vi "StandardEngineUI.vi"() -> ()   [LabVIEW 2013, in "Standard Engine Editor Node.lvclass"]
doc: "This VI creates a view for the Standard Engine Configuration class using the CEF."
uses:
  Standard Engine Editor Node.lvclass
  <vilib>/NI/Configuration Framework/Node/NodeRef.ctl
  <vilib>/NI/Configuration Framework/Node/NISE_CEF_Node.lvclass
  <vilib>/NI/AMC/Message Queue.ctl
  <vilib>/NI/AMC/Message.ctl
  <vilib>/NI/Tools/Keyed Array/KeyedArray.ctl
  <vilib>/NI/Configuration Framework/Node/UserEventRef.ctl
  <vilib>/NI/Configuration Framework/Controls/EventCluster.ctl
  Execution Engine/Configuration/Supported Timing Sources.ctl
  Processor Assignment Mode.ctl
  <vilib>/NI/Configuration Framework/Node/RefreshUIEvent.ctl
  <vilib>/NI/Configuration Framework/Node/CacheState.ctl
  <vilib>/NI/Configuration Framework/Node/StopEvent.ctl
  <vilib>/NI/Configuration Framework/Node/NodeChangeEvent.ctl
  Execution Engine/Configuration/timing reporting tags.ctl
  Execution Engine/Configuration/error options.ctl
  Execution Engine/Configuration/pre-execution timing tags.ctl
  <vilib>/Utility/miscctls.llb/LVPositionTypeDef.ctl
  <vilib>/NI/DCAF/Tag Editor Core/Configuration Editor/Classes/Engine Parent/Engine Parent Editor Node.lvclass
  Standard Engine Editor Node.lvclass/Standard Engine Editor Node.ctl
  Execution Engine/Configuration/Standard Engine Configuration.lvclass/Standard Engine Configuration.ctl
  Execution Engine/Configuration/Module Decimation.ctl
  Execution Engine/Runtime/error responses.ctl
  Execution Engine/Configuration/Write Timing Source Type.vi
  Execution Engine/Configuration/Write Master Timing Module.vi
  Execution Engine/Configuration/Write Processor.vi
  Execution Engine/Configuration/Read Processor.vi
  Execution Engine/Configuration/Read Timing Source Type.vi
  <vilib>/NI/DCAF/Tag Editor Core/Configuration Editor/Classes/Engine Parent/Read Name.vi
  <vilib>/NI/Configuration Framework/serializable configuration/get alias.vi
  Execution Engine/Configuration/Write Timing Source dt.vi
  Execution Engine/Configuration/Find Module Specific Config.vi
  <vilib>/NI/Configuration Framework/error generator/NISE_error generator.vi
  Execution Engine/Configuration/Read Timing Source dt.vi
  <vilib>/NI/DCAF UI Toolkit/Controls/DCAF UI Elements.lvlib
  Execution Engine/Configuration/Standard Engine Configuration.lvclass
  <vilib>/NI/Configuration Framework/serializable configuration/NISE_CEF_serializable configuration.lvclass
  <vilib>/NI/Tools/Keyed Array/Tools_KeyedArray.lvlib
  <vilib>/NI/AMC/AMC.lvlib
  <vilib>/NI/Configuration Framework/NISE_CEF_TreeControl.lvlib
panel:
  in  "node change":T1
  in  "stop event":T2
  in  "cache state":T3
  in  "refresh UI":T4
  in  "Tab Control":enum32{"Engine Settings", "Module Settings"}(tab)
  out "Pre-Execution Timing Tags":T5
  in  "Create Pre-Execution Timing Tags?":bool=TRUE
  in  "Create Timing Report Tags?":bool
  in  "Module Timing Source":i32(listbox)
  in  "Engine Name":string
  in  "Timing Source dt":u32=5000
  in  "Timing Source Type":T6=enum."1 kHz Clock"
  in  "Procesor Assignment":i32 min=0
  in  "Mode":T7
  in  "Warning Message":string="This timing source is not deterministic."
  out "Timing Reporting":T8={"late index (bool)"="_stdeng_late", "late count index (U32)"="_stdeng_latecount", "current dt ns(U64)"="_stdeng_iteratedt", "last exec time ns(U64)"="_stdeng_exectime"}
  in  "Offset":u16
  in  "Decimation":u16=1 min=1
  in  "Create Error Tag?":bool
  out "error tag":string
  in  "Module to Configure":i32(listbox)
  in  "Execution Order (low to high)":i32
  in  "Execute Asynchronously?":bool
  in  "Recoverable":T9
  in  "Critical":T9
  in  "Trivial":T9
  in  "Unknown":T9
  in  "user event":T10
  in  "main queue":T11
  in  "node ref":T12
  # "Processor Assignment"
  # "Timing Information"
  # "Error Actions"
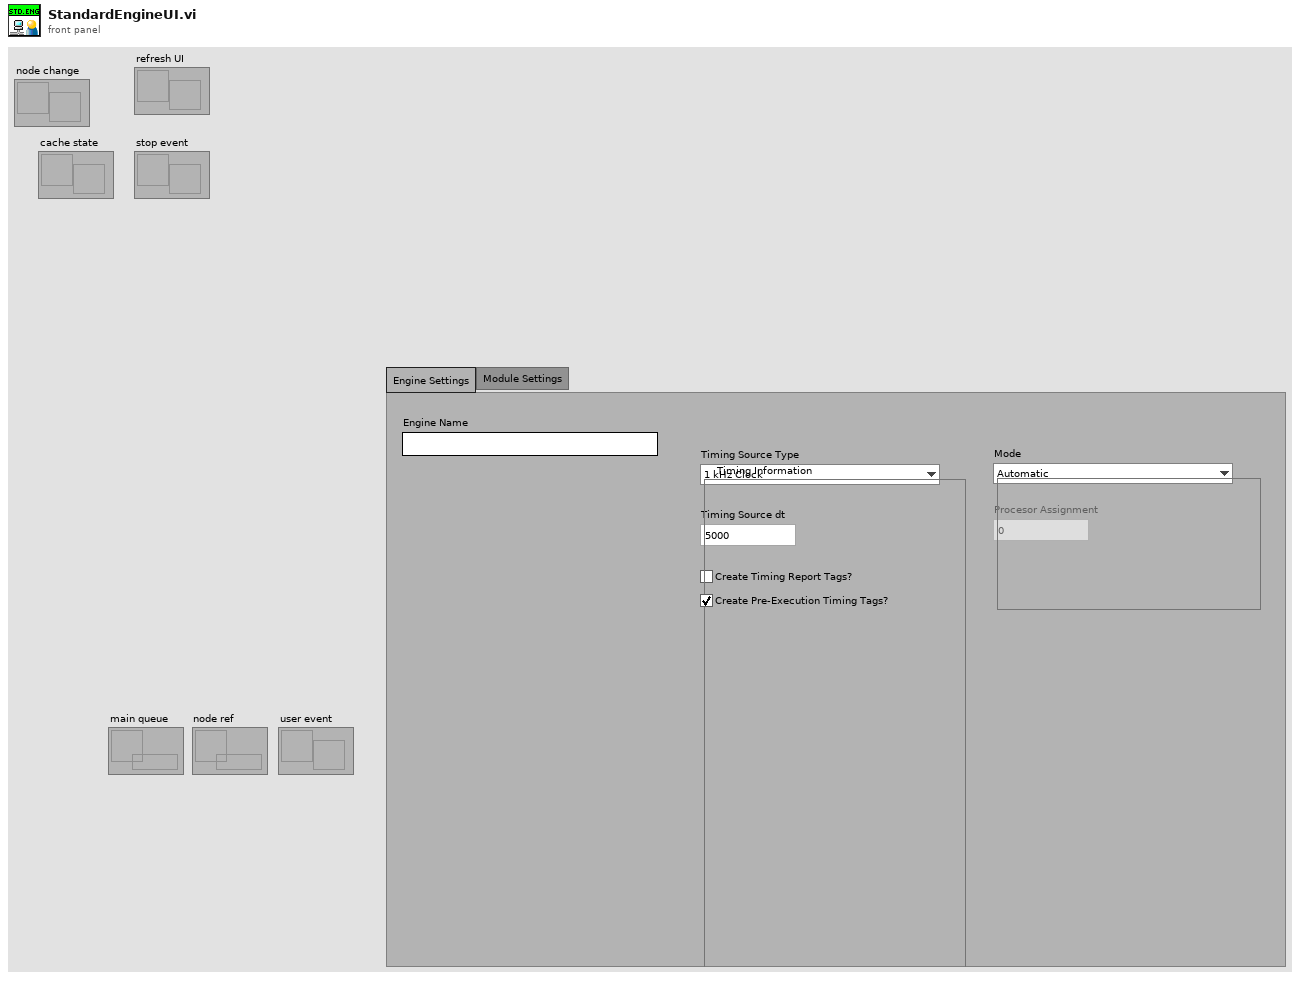
[diagram p1: front panel]
types:
  T1 = typedef "NISE_CEF_Node.lvclass/NodeChangeEvent.ctl" = refnum<user-event>
  T2 = typedef "NISE_CEF_Node.lvclass/StopEvent.ctl" = refnum<user-event>
  T3 = typedef "NISE_CEF_Node.lvclass/CacheState.ctl" = refnum<user-event>
  T4 = typedef "NISE_CEF_Node.lvclass/RefreshUIEvent.ctl" = refnum<user-event>
  T5 = typedef "Standard Engine Configuration.lvclass/pre-execution timing tags.ctl" = cluster{"iteration start seconds (DBL)":string}
  T6 = typedef "Standard Engine Configuration.lvclass/Supported Timing Sources.ctl" = enum16{"Use Module Timing Source", "1 kHz Clock", "1 MHz Clock", "Synchronize to Scan Engine"}
  T7 = typedef "Standard Engine Editor Node.lvclass/Processor Assignment Mode.ctl" = enum16{"Automatic", "Manual"}
  T8 = typedef "Standard Engine Configuration.lvclass/timing reporting tags.ctl" = cluster{"late index (bool)":string, "late count index (U32)":string, "current dt ns(U64)":string, "last exec time ns(U64)":string}
  T9 = typedef "Standard Engine Configuration.lvclass/error options.ctl" = cluster{"clear":bool, "notify":bool, "log":bool, "remove module":bool, "abort engine":bool, "go to safe state":bool, "recover module":bool}
  T10 = typedef "NISE_CEF_Node.lvclass/UserEventRef.ctl" = refnum<user-event>
  T11 = typedef "AMC.lvlib/Message Queue.ctl" = refnum<queue>
  T12 = typedef "NISE_CEF_Node.lvclass/NodeRef.ctl" = refnum<data-value>
  T13 = typedef "LVPositionTypeDef.ctl" = cluster{"Left":i32, "Top":i32}
  T14 = typedef "Standard Engine Configuration.lvclass/error responses.ctl" = cluster{"unknown":T9, "trivial":T9, "critical":T9, "recoverable":T9}
  T15 = typedef "Standard Engine Configuration.lvclass/Module Decimation.ctl" = cluster{"Decimation":u16, "Offset":u16, "sort order":i32, "async?":bool}
  T16 = enum8{"Enabled", "Disabled", "Disabled and Grayed Out"}
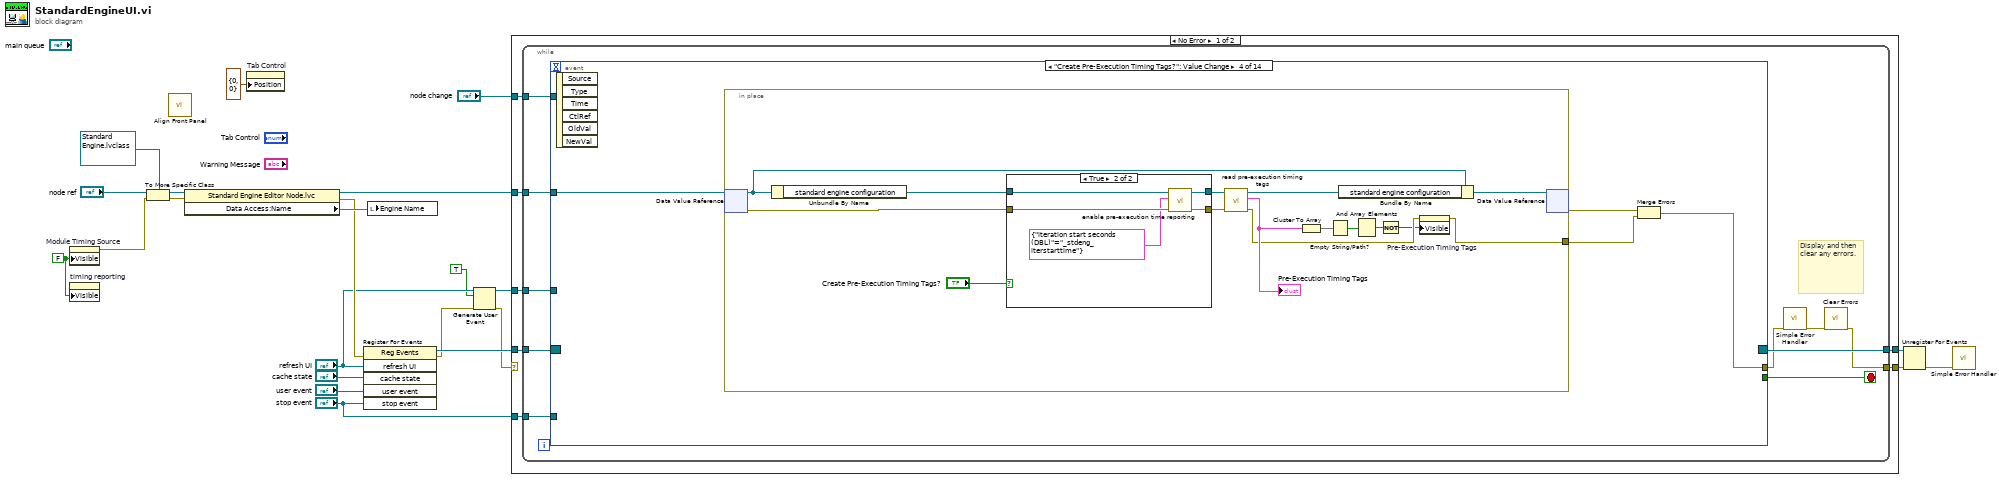
[diagram p0: block diagram]
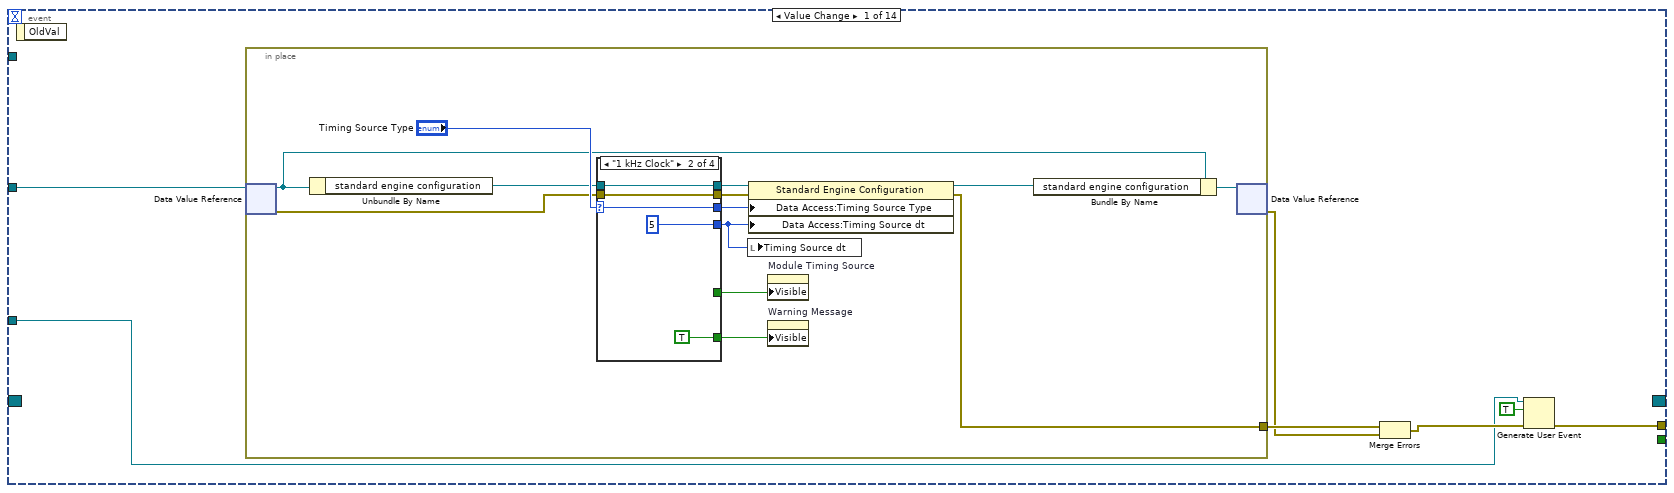
[diagram p2: hidden frame]
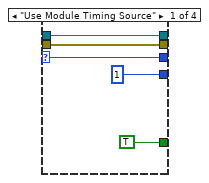
[diagram p3: hidden frame]
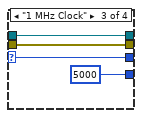
[diagram p4: hidden frame]
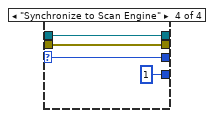
[diagram p5: hidden frame]
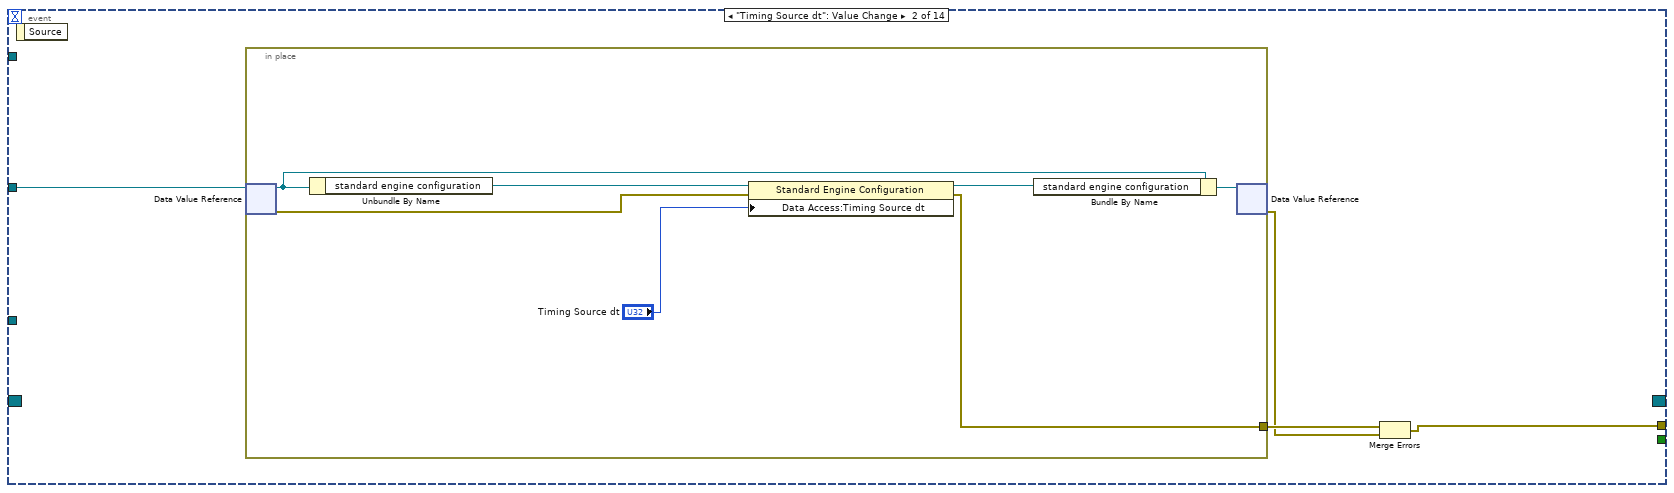
[diagram p6: hidden frame]
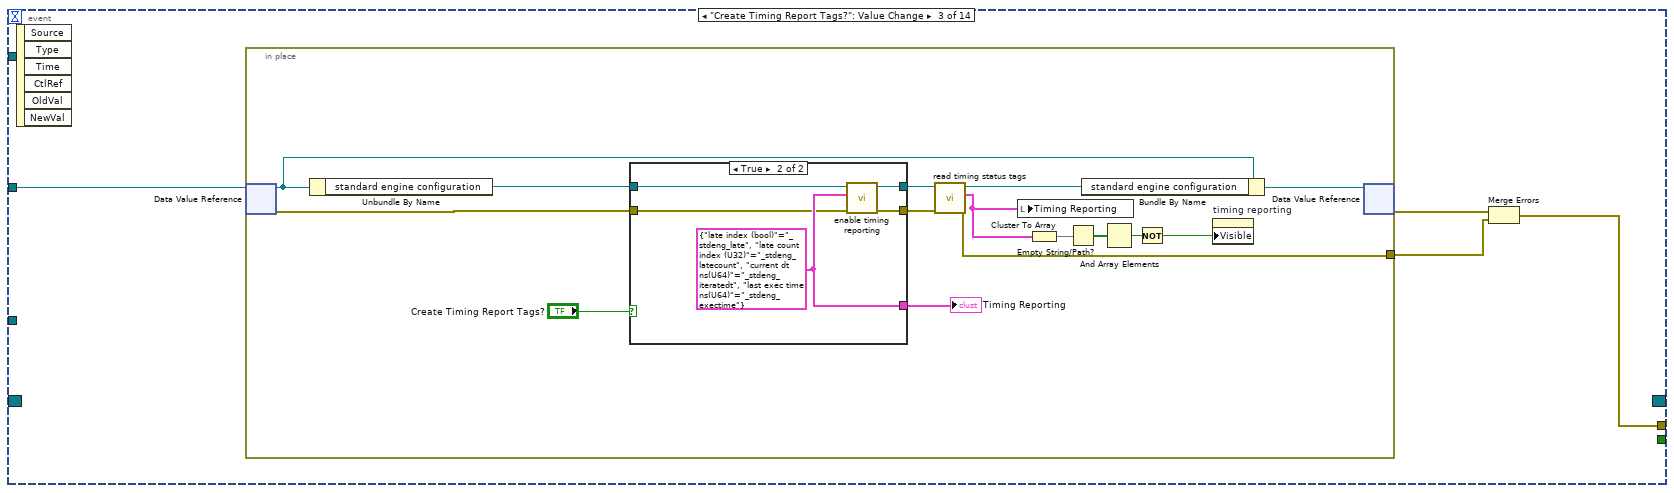
[diagram p7: hidden frame]
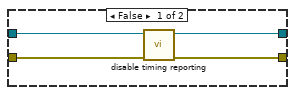
[diagram p8: hidden frame]
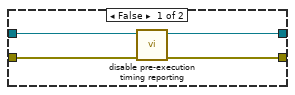
[diagram p9: hidden frame]
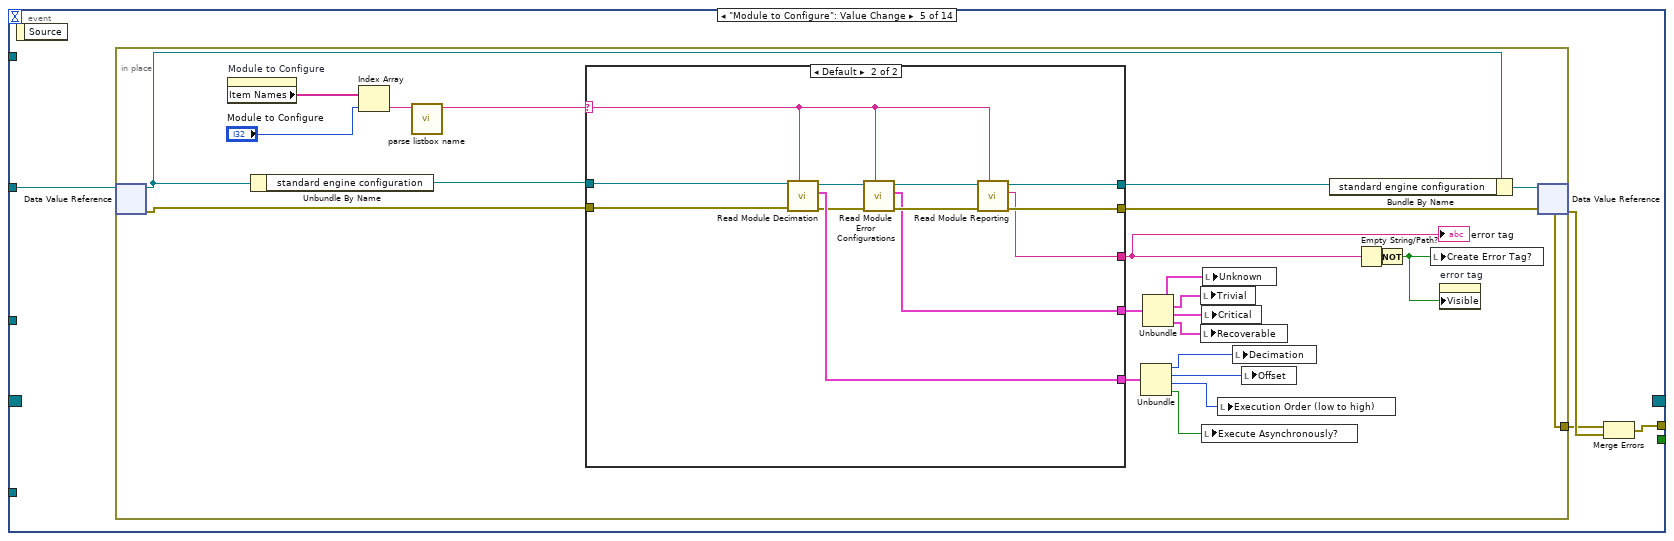
[diagram p10: hidden frame]
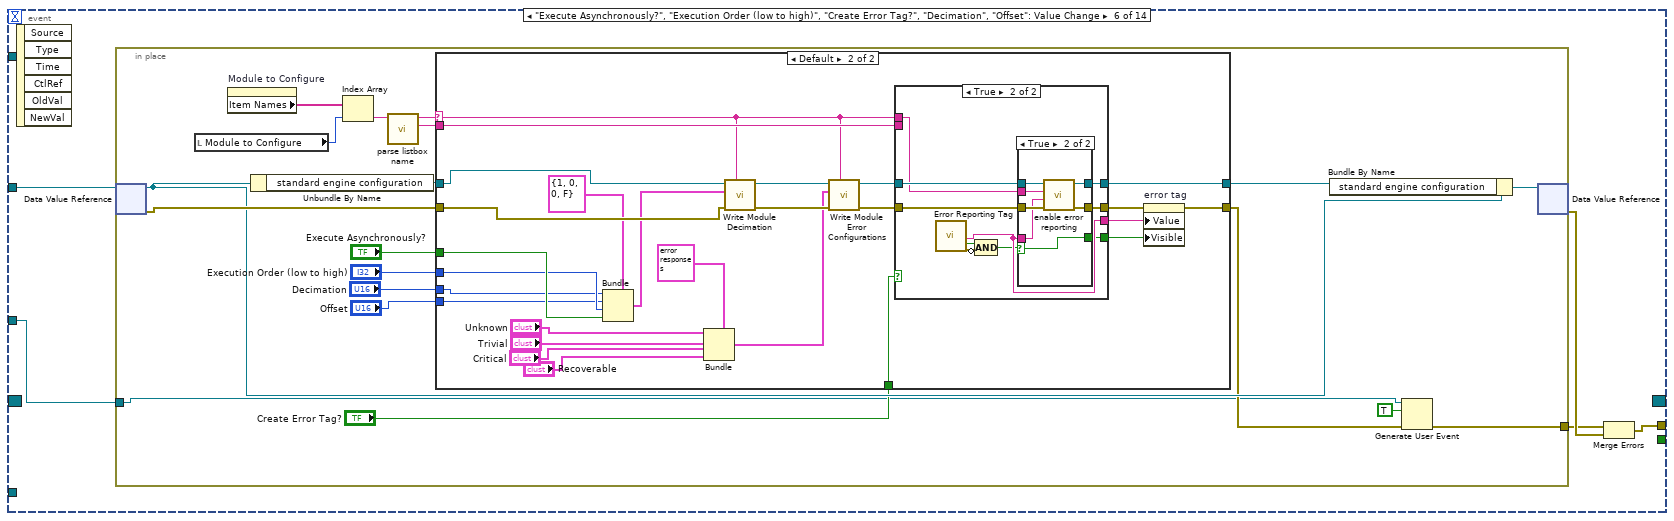
[diagram p12: hidden frame]
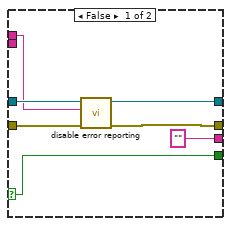
[diagram p14: hidden frame]
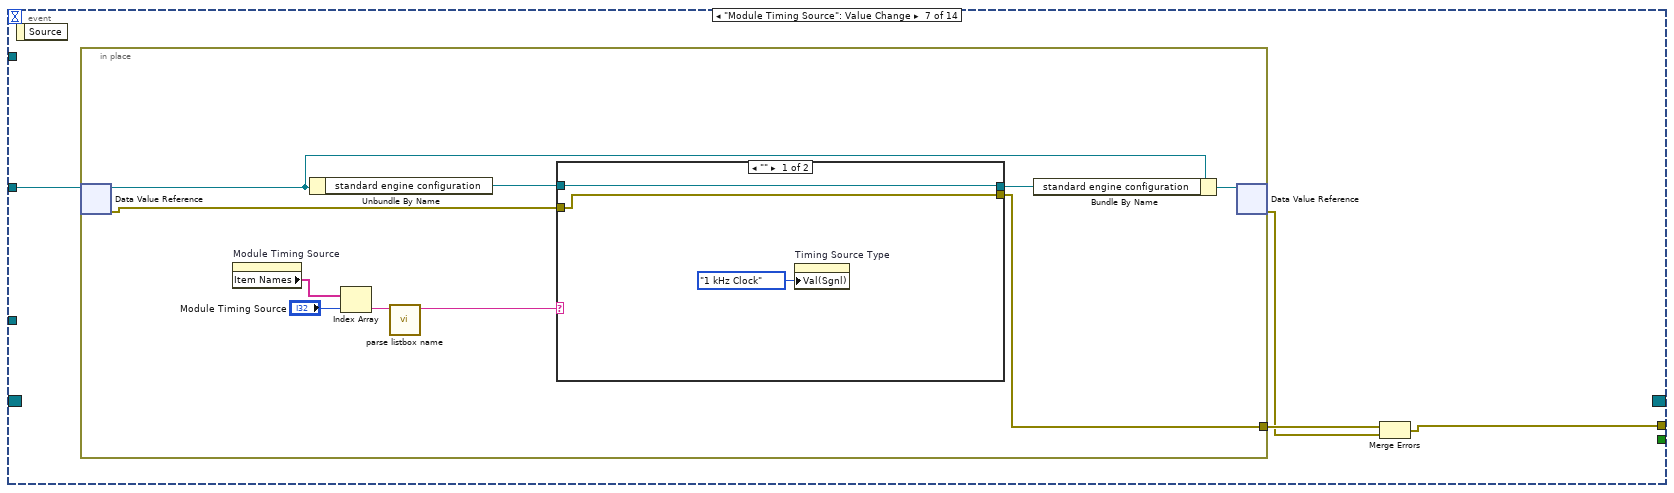
[diagram p16: hidden frame]
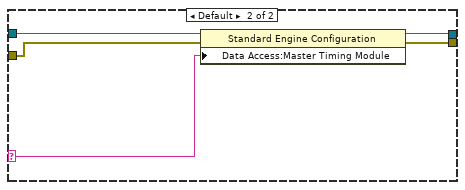
[diagram p17: hidden frame]
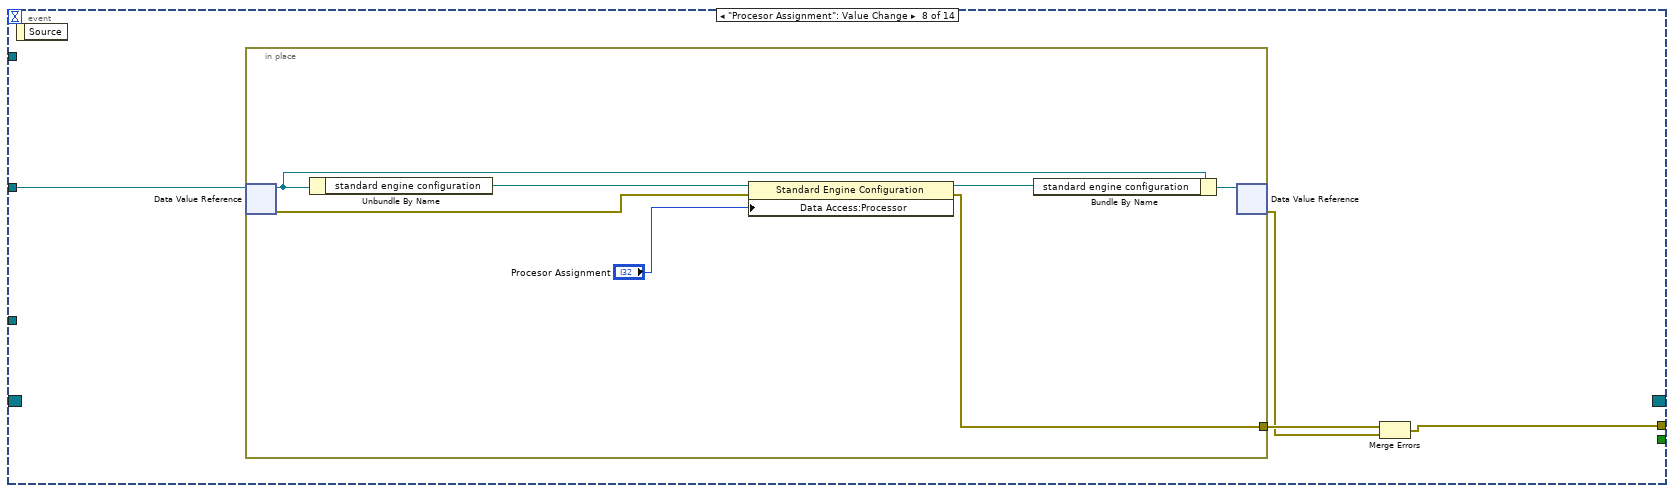
[diagram p18: hidden frame]
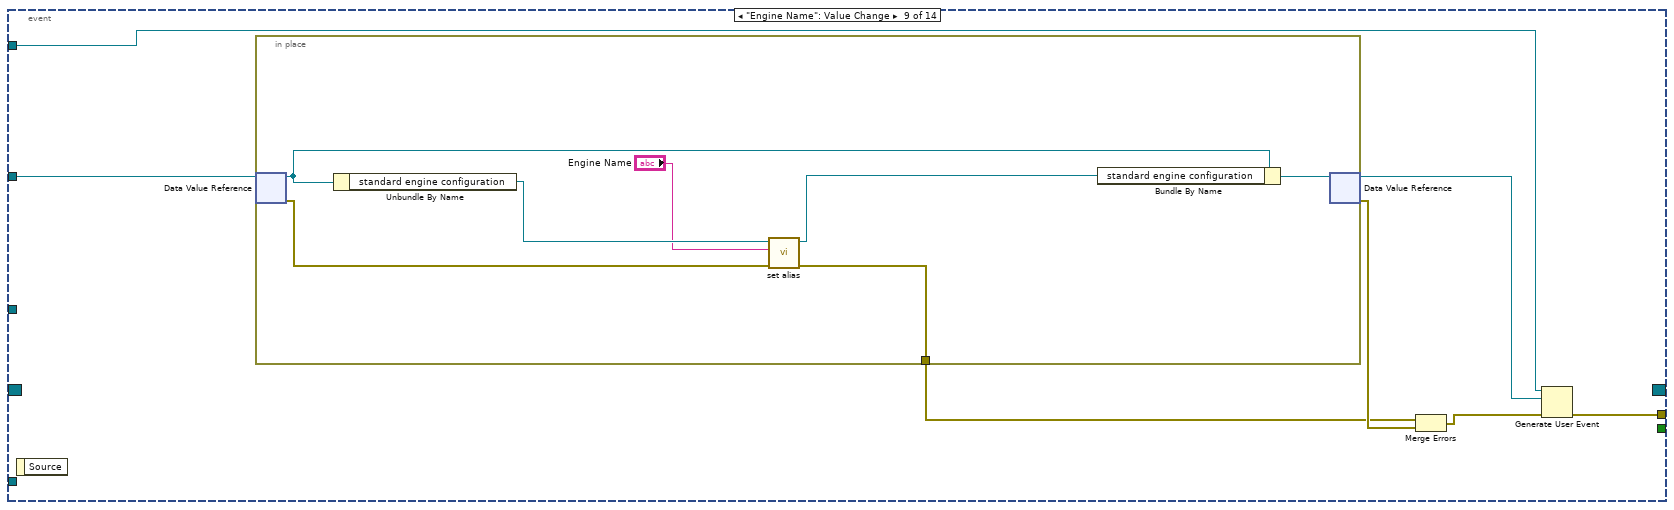
[diagram p19: hidden frame]
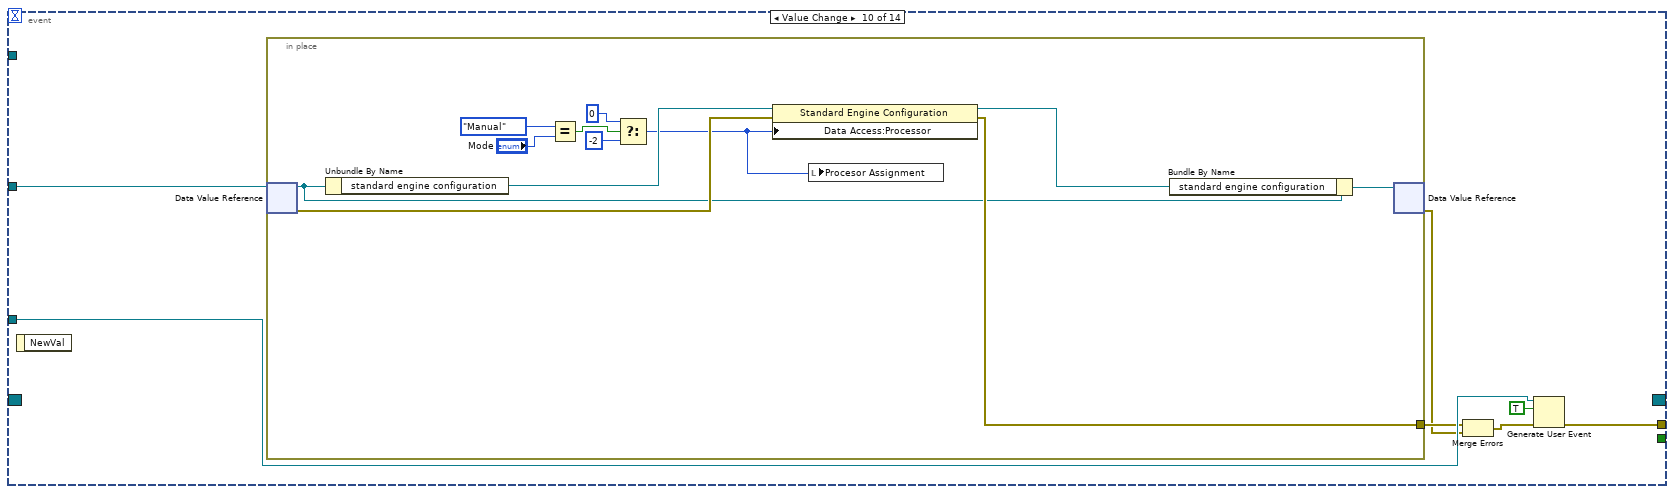
[diagram p20: hidden frame]
diagram:
  w2 = FALSE ("Visible")
  n1 = property on="Module Timing Source" class="LstBox (strict)"("Visible"=w2) -> (error out=w3:errorcluster)  [unwired: 2 in, 1 out]
  n2 = property on="timing reporting" class="Clust (strict)"("Visible"=w2) -> ()  [unwired: 2 in, 2 out]
  n3 = To More Specific Class(target class=refnum<data-value> refnum ("data value reference"), reference="node ref", error in=w3) -> (specific class reference=w19:refnum<data-value>, error out=w18:errorcluster)
  n4 = call <vilib>:"Align Front Panel.vi"() -> ()  [unwired: 10 in, 2 out]
  n5 = property class="Standard Engine Editor Node.lvc"(reference=w19, error in=w18) -> (reference out=w1:refnum<data-value>, error out=w15:errorcluster, "Data Access:Name"=w20:string)
  n6 = property on="Tab Control" class="TabCtl (strict)"("Position"=T13 {"Left"=0, "Top"=0}) -> ()  [unwired: 2 in, 2 out]
  n7 = register-events(error in=w15, "refresh UI", "cache state", "user event", "stop event") -> (reference out=w23:refnum<event-registration>, error out=w14:errorcluster)  [unwired: 1 in]
  n8 = local write "Engine Name"(w20) -> ()
  n9 = Generate User Event(user event="refresh UI", event data cluster=TRUE ("event data"), error in=w14) -> (user event out=w13:T4, error out=w6:errorcluster)  [unwired: 1 in]
  n10 = case shown="No Error" w6 {
    selector: w6 -> [_ w393]
    tunnel: w23 -> [w30 w394]
    tunnel: [w29 w394] -> w22
    tunnel: [w28 w393] -> w21
    tunnel: w1 -> [w27 _]
    tunnel: w13 -> [w26 _]
    tunnel: "stop event" -> [w25 _]
    tunnel: "node change" -> [w24 _]
    frame No Error {
      n11 = while {
        tunnel: w30 -> [w40]
        tunnel: [w39] -> w29
        tunnel: [w34] -> w28
        tunnel: w27 -> [w37]
        tunnel: w26 -> [w33]
        tunnel: w25 -> [w32]
        tunnel: w24 -> [w31]
        stop <- w38 stop-if-true
        # "Display and then clear any errors."
        n12 = event shown="[3] \"Create Pre-Execution Timing Tags?\": Value Change" {
          selector: w40 -> [_ _ _ _ _ _ _ _ _ _ _ _ _ _]
          dyn-events: [_ _ _ _ _ _ _ _ _ _ _ _ _ _] -> w39
          timeout: _ -> [_ _ _ _ _ _ _ _ _ _ _ _ _ _]
          tunnel: [_ _ _ _ _ _ _ _ _ _ w333 TRUE _ _] -> w38
          tunnel: [w43 w80 w91 w119 w148 w190 w267 w289 w301 w317 _ _ w338 _] -> w36
          tunnel: w37 -> [w46 w81 w93 w121 w149 w191 w268 w290 w305 w315 _ _ w339 _]
          tunnel: w33 -> [w42 _ _ _ _ w187 _ _ _ w319 _ _ _ _]
          tunnel: w32 -> [_ _ _ _ _ _ _ _ _ _ _ _ _ _]
          tunnel: w31 -> [_ _ _ _ _ _ _ _ w300 _ _ _ w337 _]
          event Value Change {
            n13 = event-data() -> ()  [unwired: 1 in, 1 out]
            n14 = in-place {
              in-place-border: [w57] -> w47
              n15 = in-place-dvr #1(w46) -> (w53:refnum<class "Standard Engine Editor Node.lvclass">, w55:errorcluster)
              n16 = Unbundle By Name(w53) -> ("standard engine configuration"=w54:refnum<class "Standard Engine Configuration.lvclass">)
              n17 = case shown="\"1 kHz Clock\"" "Timing Source Type" {
                selector: "Timing Source Type" -> [w65 w70 w72 w76]
                tunnel: w54 -> [w64 w69 w74 w78]
                tunnel: [w64 w69 w74 w78] -> w60
                tunnel: w55 -> [w63 w68 w73 w77]
                tunnel: [w63 w68 w73 w77] -> w59
                tunnel: [w65 w70 w72 w76] -> w56
                tunnel: [u32 1 ("Timing Source dt") u32 5 ("Timing Source dt") u32 5000 ("Timing Source dt") u32 1 ("Timing Source dt")] -> w49
                tunnel: [TRUE _ _ _] -> w50
                tunnel: [_ TRUE _ _] -> w48
                frame "Use Module Timing Source" {
                }
                frame "1 kHz Clock" {
                }
                frame "1 MHz Clock" {
                }
                frame "Synchronize to Scan Engine" {
                }
              }
              n18 = local write "Timing Source dt"(w49) -> ()
              n19 = property class="Standard Engine Configuration"(reference=w60, error in=w59, "Data Access:Timing Source Type"=w56, "Data Access:Timing Source dt"=w49) -> (reference out=w51:refnum<class "Standard Engine Configuration.lvclass">, error out=w57:errorcluster)
              n20 = property on="Module Timing Source" class="LstBox (strict)"("Visible"=w50) -> ()  [unwired: 2 in, 2 out]
              n21 = property on="Warning Message" class="Str"("Visible"=w48) -> ()  [unwired: 2 in, 2 out]
              n22 = Bundle By Name(cluster=w53, "standard engine configuration"=w51) -> (w52:refnum<class "Standard Engine Editor Node.lvclass">)
              n23 = in-place-dvr #1(w52) -> (w44:errorcluster)  [unwired: 1 out]
            }
            n24 = Merge Errors(w47, w44) -> (w45:errorcluster)
            n25 = Generate User Event(user event=w42, event data cluster=TRUE ("event data"), error in=w45) -> (error out=w43:errorcluster)  [unwired: 1 in, 1 out]
          }
          event "Timing Source dt": Value Change {
            n26 = event-data() -> ()  [unwired: 1 in, 1 out]
            n27 = in-place {
              in-place-border: [w89] -> w82
              n28 = in-place-dvr #2(w81) -> (w86:refnum<class "Standard Engine Editor Node.lvclass">, w88:errorcluster)
              n29 = Unbundle By Name(w86) -> ("standard engine configuration"=w87:refnum<class "Standard Engine Configuration.lvclass">)
              n30 = property class="Standard Engine Configuration"(reference=w87, error in=w88, "Data Access:Timing Source dt"="Timing Source dt") -> (reference out=w84:refnum<class "Standard Engine Configuration.lvclass">, error out=w89:errorcluster)
              n31 = Bundle By Name(cluster=w86, "standard engine configuration"=w84) -> (w85:refnum<class "Standard Engine Editor Node.lvclass">)
              n32 = in-place-dvr #2(w85) -> (w79:errorcluster)  [unwired: 1 out]
            }
            n33 = Merge Errors(w82, w79) -> (w80:errorcluster)
          }
          event "Create Timing Report Tags?": Value Change {
            n34 = event-data() -> ()  [unwired: 1 in, 6 out]
            n35 = in-place {
              in-place-border: [w95] -> w90
              n36 = in-place-dvr #3(w93) -> (w94:refnum<class "Standard Engine Editor Node.lvclass">, w108:errorcluster)
              n37 = Unbundle By Name(w94) -> ("standard engine configuration"=w105:refnum<class "Standard Engine Configuration.lvclass">)
              n38 = case shown="True" "Create Timing Report Tags?" {
                tunnel: w105 -> [w112 w117]
                tunnel: [w110 w116] -> w98
                tunnel: [_ w115] -> w104
                tunnel: w108 -> [w111 w114]
                tunnel: [w109 w113] -> w96
                frame False {
                  n39 = call "disable timing reporting.vi"("error in"=w111, "Standard Engine Configuration in"=w112) -> ("error out"=w109:errorcluster, "Standard Engine Configuration out"=w110:refnum<class "Standard Engine Configuration.lvclass">)  [unwired: 8 in]
                }
                frame True {
                  w115 = T8 {"late index (bool)"="_stdeng_late", "late count index (U32)"="_stdeng_latecount", "current dt ns(U64)"="_stdeng_iteratedt", "last exec time ns(U64)"="_stdeng_exectime"} ("timing reporting")
                  n40 = call "enable timing reporting.vi"("error in"=w114, "timing reporting"=w115, "Standard Engine Configuration in"=w117) -> ("error out"=w113:errorcluster, "Standard Engine Configuration out"=w116:refnum<class "Standard Engine Configuration.lvclass">)  [unwired: 7 in]
                }
              }
              "Timing Reporting" <- w104
              n41 = call "read timing status tags.vi"("error in"=w96, "Standard Engine Configuration in"=w98) -> ("error out"=w95:errorcluster, "timing reporting"=w100:T8, "Standard Engine Configuration out"=w99:refnum<class "Standard Engine Configuration.lvclass">)  [unwired: 7 in]
              n42 = local write "Timing Reporting"(w100) -> ()
              n43 = Cluster To Array(cluster=w100) -> (array=w103:string[])
              n44 = Empty String/Path?(string/path=w103) -> (empty?=w102:bool[])
              n45 = Bundle By Name(cluster=w94, "standard engine configuration"=w99) -> (w107:refnum<class "Standard Engine Editor Node.lvclass">)
              n46 = And Array Elements(Boolean array=w102) -> (logical AND=w101:bool)
              n47 = Not(x=w101) -> (.not. x?=w97:bool)
              n48 = property on="timing reporting" class="Clust (strict)"("Visible"=w97) -> ()  [unwired: 2 in, 2 out]
              n49 = in-place-dvr #3(w107) -> (w92:errorcluster)  [unwired: 1 out]
            }
            n50 = Merge Errors(w92, w90) -> (w91:errorcluster)
          }
          event "Create Pre-Execution Timing Tags?": Value Change {
            n51 = event-data() -> ()  [unwired: 1 in, 6 out]
            n52 = in-place {
              in-place-border: [w124] -> w118
              n53 = in-place-dvr #4(w121) -> (w135:refnum<class "Standard Engine Editor Node.lvclass">, w136:errorcluster)
              n54 = Unbundle By Name(w135) -> ("standard engine configuration"=w133:refnum<class "Standard Engine Configuration.lvclass">)
              n55 = case shown="True" "Create Pre-Execution Timing Tags?" {
                tunnel: w133 -> [w139 w145]
                tunnel: [w138 w144] -> w128
                tunnel: w136 -> [w140 w143]
                tunnel: [w137 w142] -> w126
                frame False {
                  n56 = call "disable pre-execution timing reporting.vi"("error in"=w140, "Standard Engine Configuration in"=w139) -> ("error out"=w137:errorcluster, "Standard Engine Configuration out"=w138:refnum<class "Standard Engine Configuration.lvclass">)  [unwired: 8 in]
                }
                frame True {
                  n57 = call "enable pre-execution time reporting.vi"("error in"=w143, "pre-execution timing tags"=T5 {"iteration start seconds (DBL)"="_stdeng_iterstarttime"}, "Standard Engine Configuration in"=w145) -> ("error out"=w142:errorcluster, "Standard Engine Configuration out"=w144:refnum<class "Standard Engine Configuration.lvclass">)  [unwired: 7 in]
                }
              }
              n58 = call "read pre-execution timing tags.vi"("error in"=w126, "Standard Engine Configuration in"=w128) -> ("error out"=w123:errorcluster, "pre-execution timing tags"=w125:T5, "Standard Engine Configuration out"=w127:refnum<class "Standard Engine Configuration.lvclass">)  [unwired: 7 in]
              "Pre-Execution Timing Tags" <- w125
              n59 = Cluster To Array(cluster=w125) -> (array=w132:string[])
              n60 = Empty String/Path?(string/path=w132) -> (empty?=w131:bool[])
              n61 = Bundle By Name(cluster=w135, "standard engine configuration"=w127) -> (w134:refnum<class "Standard Engine Editor Node.lvclass">)
              n62 = And Array Elements(Boolean array=w131) -> (logical AND=w130:bool)
              n63 = Not(x=w130) -> (.not. x?=w122:bool)
              n64 = property on="Pre-Execution Timing Tags" class="Clust (strict)"(error in=w123, "Visible"=w122) -> (error out=w124:errorcluster)  [unwired: 1 in, 1 out]
              n65 = in-place-dvr #4(w134) -> (w120:errorcluster)  [unwired: 1 out]
            }
            n66 = Merge Errors(w120, w118) -> (w119:errorcluster)
          }
          event "Module to Configure": Value Change {
            n67 = event-data() -> ()  [unwired: 1 in, 1 out]
            n68 = in-place {
              in-place-border: [w164] -> w146
              n69 = in-place-dvr #5(w149) -> (w171:refnum<class "Standard Engine Editor Node.lvclass">, w172:errorcluster)
              n70 = property on="Module to Configure" class="LstBox (strict)"() -> ("Item Names"=w169:string[])  [unwired: 2 in, 2 out]
              n71 = Unbundle By Name(w171) -> ("standard engine configuration"=w166:refnum<class "Standard Engine Configuration.lvclass">)
              n72 = Index Array(array=w169, index="Module to Configure") -> (element=w167:string)
              n73 = call "parse listbox name.vi"("formatted name"=w167) -> ("ID"=w160:string)  [unwired: 9 in, 1 out]
              n74 = case shown="Default" w160 {
                selector: w160 -> [_ w176]
                tunnel: w166 -> [w174 w186]
                tunnel: w172 -> [w173 w185]
                tunnel: [_ w184] -> w159
                tunnel: [w173 w179] -> w164
                tunnel: [w174 w178] -> w163
                tunnel: [_ w177] -> w162
                tunnel: [_ w175] -> w154
                frame "" {
                }
                frame Default {
                  n75 = call "Read Module Decimation.vi"("Module ID"=w176, "error in"=w185, "Standard Engine Repo Data in"=w186) -> ("error out"=w182:errorcluster, "Module Decimation"=w184:T15, "Standard Engine Repo Data out"=w183:refnum<class "Standard Engine Configuration.lvclass">)  [unwired: 6 in]
                  n76 = call "Read Module Error Configurations.vi"("Module ID"=w176, "error in"=w182, "Standard Engine Repo Data in"=w183) -> ("error out"=w180:errorcluster, "error responses"=w175:T14, "Standard Engine Repo Data out"=w181:refnum<class "Standard Engine Configuration.lvclass">)  [unwired: 6 in]
                  n77 = call "Read Module Reporting.vi"("Module ID"=w176, "error in"=w180, "Standard Engine Repo Data in"=w181) -> ("error out"=w179:errorcluster, "error tag"=w177:string, "Standard Engine Repo Data out"=w178:refnum<class "Standard Engine Configuration.lvclass">)  [unwired: 6 in]
                }
              }
              "error tag" <- w162
              n78 = Unbundle(w159) -> ("Decimation"=w155:u16, "Offset"=w156:u16, "sort order"=w157:i32, "async?"=w158:bool)
              n79 = Unbundle(w154) -> ("unknown"=w150:T9, "trivial"=w151:T9, "critical"=w152:T9, "recoverable"=w153:T9)
              n80 = local write "Trivial"(w151) -> ()
              n81 = local write "Recoverable"(w153) -> ()
              n82 = local write "Critical"(w152) -> ()
              n83 = local write "Execute Asynchronously?"(w158) -> ()
              n84 = local write "Unknown"(w150) -> ()
              n85 = local write "Execution Order (low to high)"(w157) -> ()
              n86 = local write "Decimation"(w155) -> ()
              n87 = local write "Offset"(w156) -> ()
              n88 = Bundle By Name(cluster=w171, "standard engine configuration"=w163) -> (w170:refnum<class "Standard Engine Editor Node.lvclass">)
              n89 = Empty String/Path?(string/path=w162) -> (empty?=w165:bool)
              n90 = Not(x=w165) -> (.not. x?=w161:bool)
              n91 = local write "Create Error Tag?"(w161) -> ()
              n92 = property on="error tag" class="Str"("Visible"=w161) -> ()  [unwired: 2 in, 2 out]
              n93 = in-place-dvr #5(w170) -> (w147:errorcluster)  [unwired: 1 out]
            }
            n94 = Merge Errors(w146, w147) -> (w148:errorcluster)
          }
          event "Execute Asynchronously?", "Execution Order (low to high)", "Create Error Tag?", "Decimation", "Offset": Value Change {
            n95 = event-data() -> ()  [unwired: 1 in, 6 out]
            n96 = in-place {
              in-place-border: [w196] -> w188
              in-place-border: w187 -> [w195]
              n97 = in-place-dvr #6(w191) -> (w209:refnum<class "Standard Engine Editor Node.lvclass">, w210:errorcluster)
              n98 = local read "Module to Configure"() -> (w202:i32)
              n99 = property on="Module to Configure" class="LstBox (strict)"() -> ("Item Names"=w207:string[])  [unwired: 2 in, 2 out]
              n100 = Unbundle By Name(w209) -> ("standard engine configuration"=w205:refnum<class "Standard Engine Configuration.lvclass">)
              n101 = Index Array(array=w207, index=w202) -> (element=w206:string)
              n102 = call "parse listbox name.vi"("formatted name"=w206) -> ("display"=w198:string, "ID"=w197:string)  [unwired: 9 in]
              n103 = case shown="Default" w197 {
                selector: w197 -> [_ w226]
                tunnel: w205 -> [w212 w238]
                tunnel: w210 -> [w211 w237]
                tunnel: "Execute Asynchronously?" -> [_ w222]
                tunnel: "Execution Order (low to high)" -> [_ w221]
                tunnel: [w212 w232] -> w201
                tunnel: [w211 w231] -> w200
                tunnel: "Create Error Tag?" -> [_ w229]
                tunnel: w198 -> [_ w227]
                tunnel: "Decimation" -> [_ w220]
                tunnel: "Offset" -> [_ w219]
                frame "" {
                }
                frame Default {
                  n104 = Bundle(cluster=T15 {"Decimation"=1, "Offset"=0, "sort order"=0, "async?"=FALSE} ("Module Decimation"), "Decimation"=w220, "Offset"=w219, "sort order"=w221, "async?"=w222) -> (w223:T15)
                  n105 = Bundle(cluster=T14 {"unknown"={"clear"=FALSE, "notify"=FALSE, "log"=FALSE, "remove module"=FALSE, "abort engine"=FALSE, "go to safe state"=FALSE, "recover module"=FALSE}, "trivial"={"clear"=FALSE, "notify"=FALSE, "log"=FALSE, "remove module"=FALSE, "abort engine"=FALSE, "go to safe state"=FALSE, "recover module"=FALSE}, "critical"={"clear"=FALSE, "notify"=FALSE, "log"=FALSE, "remove module"=FALSE, "abort engine"=FALSE, "go to safe state"=FALSE, "recover module"=FALSE}, "recoverable"={"clear"=FALSE, "notify"=FALSE, "log"=FALSE, "remove module"=FALSE, "abort engine"=FALSE, "go to safe state"=FALSE, "recover module"=FALSE}} ("error responses"), "unknown"="Unknown", "trivial"="Trivial", "critical"="Critical", "recoverable"="Recoverable") -> (w217:T14)
                  n106 = call "Write Module Decimation.vi"("Module ID"=w226, "error in"=w237, "Module Decimation"=w223, "Standard Engine Repo Data in"=w238) -> ("error out"=w235:errorcluster, "Standard Engine Repo Data out"=w236:refnum<class "Standard Engine Configuration.lvclass">)  [unwired: 6 in]
                  n107 = call "Write Module Error Configurations.vi"("Module ID"=w226, "error in"=w235, "error responses"=w217, "Standard Engine Repo Data in"=w236) -> ("error out"=w233:errorcluster, "Standard Engine Repo Data out"=w234:refnum<class "Standard Engine Configuration.lvclass">)  [unwired: 6 in]
                  n108 = case shown="True" w229 {
                    selector: w229 -> [w239 _]
                    tunnel: w234 -> [w245 w255]
                    tunnel: w233 -> [w244 w254]
                    tunnel: [w242 w253] -> w232
                    tunnel: [w243 w252] -> w230
                    tunnel: w226 -> [w241 w251]
                    tunnel: ["" w250] -> w228
                    tunnel: w227 -> [_ _]
                    tunnel: [w239 w246] -> w225
                    frame False {
                      n109 = call "disable error reporting.vi"("error in"=w244, "module ID"=w241, "Standard Engine Configuration in"=w245) -> ("error out"=w243:errorcluster, "Standard Engine Configuration out"=w242:refnum<class "Standard Engine Configuration.lvclass">)  [unwired: 7 in]
                    }
                    frame True {
                      n110 = call "Error Reporting Tag"() -> ("Tag Name"=w250:string, "OK"=w249:bool, "error out"=w248:errorcluster)  [unwired: 17 in]
                      n111 = Compound Arithmetic op=AND(w249, invert w248) -> (w247:bool)
                      n112 = case shown="True" w247 {
                        selector: w247 -> [w256 w259]
                        tunnel: w255 -> [w258 w265]
                        tunnel: w254 -> [w257 w264]
                        tunnel: [w258 w263] -> w253
                        tunnel: [w257 w262] -> w252
                        tunnel: w251 -> [_ w261]
                        tunnel: w250 -> [_ w260]
                        tunnel: [w256 w259] -> w246
                        frame False {
                        }
                        frame True {
                          n113 = call "enable error reporting.vi"("error in"=w264, "tag"=w260, "module ID"=w261, "Standard Engine Configuration in"=w265) -> ("error out"=w262:errorcluster, "Standard Engine Configuration out"=w263:refnum<class "Standard Engine Configuration.lvclass">)  [unwired: 6 in]
                        }
                      }
                    }
                  }
                  n114 = property on="error tag" class="Str"(error in=w230, "Value"=w228, "Visible"=w225) -> (error out=w231:errorcluster)  [unwired: 1 in, 1 out]
                }
              }
              n115 = Bundle By Name(cluster=w209, "standard engine configuration"=w201) -> (w208:refnum<class "Standard Engine Editor Node.lvclass">)
              n116 = Generate User Event(user event=w195, event data cluster=TRUE ("event data"), error in=w200) -> (error out=w196:errorcluster)  [unwired: 1 in, 1 out]
              n117 = in-place-dvr #6(w208) -> (w189:errorcluster)  [unwired: 1 out]
            }
            n118 = Merge Errors(w188, w189) -> (w190:errorcluster)
          }
          event "Module Timing Source": Value Change {
            n119 = event-data() -> ()  [unwired: 1 in, 1 out]
            n120 = in-place {
              in-place-border: [w279] -> w269
              n121 = in-place-dvr #7(w268) -> (w276:refnum<class "Standard Engine Editor Node.lvclass">, w278:errorcluster)
              n122 = property on="Module Timing Source" class="LstBox (strict)"() -> ("Item Names"=w272:string[])  [unwired: 2 in, 2 out]
              n123 = Unbundle By Name(w276) -> ("standard engine configuration"=w277:refnum<class "Standard Engine Configuration.lvclass">)
              n124 = Index Array(array=w272, index="Module Timing Source") -> (element=w271:string)
              n125 = call "parse listbox name.vi"("formatted name"=w271) -> ("ID"=w270:string)  [unwired: 9 in, 1 out]
              n126 = case shown="\"\"" w270 {
                selector: w270 -> [_ w283]
                tunnel: [w282 w287] -> w279
                tunnel: w278 -> [w282 w286]
                tunnel: w277 -> [w281 w285]
                tunnel: [w281 w284] -> w274
                frame "" {
                  n127 = property on="Timing Source Type" class="Enum (strict)"("Val(Sgnl)"=Supported_Timing_Sources."1 kHz Clock" ("Value (Signaling)")) -> ()  [unwired: 2 in, 2 out]
                }
                frame Default {
                  n128 = property class="Standard Engine Configuration"(reference=w285, error in=w286, "Data Access:Master Timing Module"=w283) -> (reference out=w284:refnum<class "Standard Engine Configuration.lvclass">, error out=w287:errorcluster)
                }
              }
              n129 = Bundle By Name(cluster=w276, "standard engine configuration"=w274) -> (w275:refnum<class "Standard Engine Editor Node.lvclass">)
              n130 = in-place-dvr #7(w275) -> (w266:errorcluster)  [unwired: 1 out]
            }
            n131 = Merge Errors(w269, w266) -> (w267:errorcluster)
          }
          event "Procesor Assignment": Value Change {
            n132 = event-data() -> ()  [unwired: 1 in, 1 out]
            n133 = in-place {
              in-place-border: [w298] -> w291
              n134 = in-place-dvr #8(w290) -> (w295:refnum<class "Standard Engine Editor Node.lvclass">, w297:errorcluster)
              n135 = Unbundle By Name(w295) -> ("standard engine configuration"=w296:refnum<class "Standard Engine Configuration.lvclass">)
              n136 = property class="Standard Engine Configuration"(reference=w296, error in=w297, "Data Access:Processor"="Procesor Assignment") -> (reference out=w293:refnum<class "Standard Engine Configuration.lvclass">, error out=w298:errorcluster)
              n137 = Bundle By Name(cluster=w295, "standard engine configuration"=w293) -> (w294:refnum<class "Standard Engine Editor Node.lvclass">)
              n138 = in-place-dvr #8(w294) -> (w288:errorcluster)  [unwired: 1 out]
            }
            n139 = Merge Errors(w291, w288) -> (w289:errorcluster)
          }
          event "Engine Name": Value Change {
            n140 = event-data() -> ()  [unwired: 1 in, 1 out]
            n141 = in-place {
              in-place-border: [w309] -> w303
              n142 = in-place-dvr #9(w305) -> (w312:refnum<class "Standard Engine Editor Node.lvclass">, w310:errorcluster)
              n143 = Unbundle By Name(w312) -> ("standard engine configuration"=w307:refnum<class "Standard Engine Configuration.lvclass">)
              n144 = call <vilib>:"set alias.vi"("error in"=w310, "alias"="Engine Name", "configuration in"=w307) -> ("error out"=w309:errorcluster, "configuration out"=w308:refnum<class "Standard Engine Configuration.lvclass">)  [unwired: 7 in]
              n145 = Bundle By Name(cluster=w312, "standard engine configuration"=w308) -> (w311:refnum<class "Standard Engine Editor Node.lvclass">)
              n146 = in-place-dvr #9(w311) -> (w299:refnum<data-value>, w304:errorcluster)
            }
            n147 = Merge Errors(w303, w304) -> (w302:errorcluster)
            n148 = Generate User Event(user event=w300, event data cluster=w299, error in=w302) -> (error out=w301:errorcluster)  [unwired: 1 in, 1 out]
          }
          event Value Change {
            n149 = event-data() -> ()  [unwired: 1 in, 1 out]
            n150 = in-place {
              in-place-border: [w327] -> w318
              n151 = in-place-dvr #10(w315) -> (w325:refnum<class "Standard Engine Editor Node.lvclass">, w326:errorcluster)
              n152 = Unbundle By Name(w325) -> ("standard engine configuration"=w322:refnum<class "Standard Engine Configuration.lvclass">)
              n153 = Equal?(x=Processor_Assignment_Mode."Manual", y="Mode") -> (x = y?=w328:bool)
              n154 = Select(t=0, s=w328, f=-2 ("Processor")) -> (s? t:f=w321:i32)
              n155 = property class="Standard Engine Configuration"(reference=w322, error in=w326, "Data Access:Processor"=w321) -> (reference out=w323:refnum<class "Standard Engine Configuration.lvclass">, error out=w327:errorcluster)
              n156 = local write "Procesor Assignment"(w321) -> ()
              n157 = Bundle By Name(cluster=w325, "standard engine configuration"=w323) -> (w324:refnum<class "Standard Engine Editor Node.lvclass">)
              n158 = in-place-dvr #10(w324) -> (w314:errorcluster)  [unwired: 1 out]
            }
            n159 = Merge Errors(w318, w314) -> (w316:errorcluster)
            n160 = Generate User Event(user event=w319, event data cluster=TRUE ("event data"), error in=w316) -> (error out=w317:errorcluster)  [unwired: 1 in, 1 out]
          }
          event User Event {
            n161 = event-data() -> ("command"=w332:string)  [unwired: 1 in, 1 out]
            n162 = case shown="\"Stop\"" w332 {
              tunnel: [_ TRUE] -> w333
              frame Default {
              }
              frame "Stop" {
              }
            }
          }
          event User Event {
            n163 = event-data() -> ()  [unwired: 1 in, 1 out]
          }
          event User Event {
            n164 = event-data() -> ()  [unwired: 1 in, 5 out]
            n165 = call "Get Child Info.vi"("Data Value Reference in"=w339) -> ("error out"=w336:errorcluster, "Instance Identifier"=w340:string[], "Display Names"=w341:string[])  [unwired: 8 in]
            n166 = case shown="No Error" w336 {
              tunnel: w341 -> [w353 _]
              tunnel: w340 -> [w352 _]
              tunnel: w339 -> [w351 _]
              tunnel: [w350 errorcluster {"status"=FALSE, "code"=0, "source"=""} ("error IO")] -> w338
              tunnel: w337 -> [w343 _]
              frame No Error {
                n167 = in-place {
                  in-place-border: [w391] -> w354
                  in-place-border: w353 -> [w390]
                  in-place-border: w352 -> [w389]
                  n168 = in-place-dvr #11(w351) -> (w385:refnum<class "Standard Engine Editor Node.lvclass">, w384:errorcluster)
                  n169 = Unbundle(w385) -> (w388:refnum<class "Standard Engine Configuration.lvclass">)
                  n170 = call "Update Configuration with Existing Modules.vi"("Module IDs"=w389, "error in"=w384, "Standard Engine Configuration in"=w388) -> ("error out"=w362:errorcluster, "Standard Engine Configuration out"=w361:refnum<class "Standard Engine Configuration.lvclass">)  [unwired: 7 in]
                  n171 = call "read pre-execution timing tags.vi"("error in"=w362, "Standard Engine Configuration in"=w361) -> ("error out"=w359:errorcluster, "pre-execution timing tags"=w357:T5, "Standard Engine Configuration out"=w360:refnum<class "Standard Engine Configuration.lvclass">)  [unwired: 7 in]
                  n172 = Cluster To Array(cluster=w357) -> (array=w365:string[])
                  n173 = Empty String/Path?(string/path=w365) -> (empty?=w364:bool[])
                  n174 = Or Array Elements(Boolean array=w364) -> (logical OR=w363:bool)
                  n175 = Not(x=w363) -> (.not. x?=w358:bool)
                  n176 = local write "Create Pre-Execution Timing Tags?"(w358) -> ()
                  n177 = call "read timing status tags.vi"("error in"=w359, "Standard Engine Configuration in"=w360) -> ("error out"=w374:errorcluster, "timing reporting"=w366:T8, "Standard Engine Configuration out"=w375:refnum<class "Standard Engine Configuration.lvclass">)  [unwired: 7 in]
                  n178 = local read "Module to Configure"() -> (w376:i32)
                  n179 = local write "Timing Reporting"(w366) -> ()
                  n180 = Cluster To Array(cluster=w366) -> (array=w373:string[])
                  n181 = call "create module list.vi"("Instance Identifier"=w389, "Display Names"=w390) -> ("listbox names"=w377:string[])  [unwired: 9 in]
                  n182 = property class="Standard Engine Configuration"(reference=w375, error in=w374) -> (reference out=w386:refnum<class "Standard Engine Configuration.lvclass">, error out=w391:errorcluster, "Data Access:Timing Source dt"=w378:u32, "Data Access:Processor"=w379:i32, "Data Access:Timing Source Type"=w369:T6)
                  n183 = Empty String/Path?(string/path=w373) -> (empty?=w372:bool[])
                  n184 = And Array Elements(Boolean array=w372) -> (logical AND=w371:bool)
                  n185 = property on="Module to Configure" class="LstBox (strict)"("Item Names"=w377, "Val(Sgnl)"=w376) -> ()  [unwired: 2 in, 2 out]
                  n186 = property on="Module Timing Source" class="LstBox (strict)"("Item Names"=w377) -> ()  [unwired: 2 in, 2 out]
                  n187 = Not(x=w371) -> (.not. x?=w370:bool)
                  n188 = local write "Create Timing Report Tags?"(w370) -> ()
                  n189 = call "Processor Assignment Display.vi"("Data Access:Processor"=w379) -> ("Enabled?"=w381:T16, "Mode"=w380:T7)  [unwired: 9 in]
                  n190 = Equal?(x=w369, y=Supported_Timing_Sources."Use Module Timing Source") -> (x = y?=w367:bool)
                  n191 = local write "Procesor Assignment"(w379) -> ()
                  n192 = local write "Timing Source Type"(w369) -> ()
                  n193 = local write "Timing Source dt"(w378) -> ()
                  n194 = property on="Module Timing Source" class="LstBox (strict)"("Visible"=w367) -> ()  [unwired: 2 in, 2 out]
                  n195 = local write "Mode"(w380) -> ()
                  n196 = property on="Procesor Assignment" class="DigNum (strict)"("DisabledEnum"=w381) -> ()  [unwired: 2 in, 2 out]
                  n197 = Equal?(x=Supported_Timing_Sources."1 kHz Clock" ("Timing Source Type"), y=w369) -> (x = y?=w382:bool)
                  n198 = Bundle(cluster=w385, w386) -> (w387:refnum<class "Standard Engine Editor Node.lvclass">)
                  n199 = property on="Warning Message" class="Str"("Visible"=w382) -> ()  [unwired: 2 in, 2 out]
                  n200 = in-place-dvr #11(w387) -> (w344:refnum<data-value>, w349:errorcluster)
                }
                n201 = Get Date/Time In Seconds() -> (seconds since 1Jan1904=w347:timestamp)
                n202 = feedback #12(w347) -> (w348:timestamp)
                n203 = feedback-in #12(w347) -> ()
                n204 = Subtract(x=w347, y=w348) -> (x-y=w346:dbl)
                n205 = Greater?(x=w346, y=10.0) -> (0:w342:bool)
                n206 = case shown="True" w342 {
                  tunnel: w344 -> [_ w355]
                  tunnel: w343 -> [_ w356]
                  frame False {
                  }
                  frame True {
                    n207 = Generate User Event(user event=w356, event data cluster=w355) -> ()  [unwired: 2 in, 2 out]
                  }
                }
                n208 = Merge Errors(w354, w349) -> (w350:errorcluster)
              }
              frame Error {
              }
            }
          }
          event User Event {
            n209 = event-data() -> ()  [unwired: 1 in, 5 out]
          }
        }
        n210 = call <vilib>:"Simple Error Handler.vi"("error in (no error)"=w36) -> ("error out"=w35:errorcluster)  [unwired: 4 in, 4 out]
        n211 = call <vilib>:"Clear Errors.vi"("error in (no error)"=w35) -> ("error out"=w34:errorcluster)  [unwired: 6 in]
      }
    }
    frame Error {
    }
  }
  n212 = Unregister For Events(event registration refnum=w22, error in=w21) -> (error out=w17:errorcluster)
  n213 = call <vilib>:"Simple Error Handler.vi"("error in (no error)"=w17) -> ()  [unwired: 4 in, 5 out]
